vi "SetOccurrence.vi"(11 "occurence":i32) -> ()   [LabVIEW 2011]
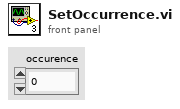
[diagram p1: front panel]
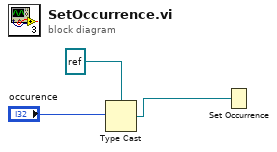
[diagram p0: block diagram]
diagram:
  n1 = Type Cast(type=refnum<k4> refnum ("事件发生"), x="occurence") -> (*(type *) &x=w1:refnum<k4>)
  n2 = Set Occurrence(w1) -> ()
